vi "Global Variables.vi"() -> ()   [LabVIEW 2017]
uses:
  GRIP Contours Report.ctl
panel:
  out "Oh Crap":bool
  in  "Intake Motor Power":dbl
  in  "Intake Angle Setpoint":dbl
  in  "Intake Angle Encoder":dbl
  out "Linear Actuator Setpoint":dbl=0.6
  out "Climb?":bool
  out "Drive Gear":enum16{"Low", "High"}(ring)
  out "Elevator Gear":enum16{"Low", "High"}(ring)=enum."High"
  out "Elevator Angle":T1(ring)
  out "Elevator Position":T2(ring)
  out "Intake Hinge Position":enum16{"Up", "Down"}(ring)
  out "Setpoint":dbl=0.5
  out "Intake State":enum16{"Off", "Intake", "Spit Low", "Spit High"}(ring)
  out "Power Cube Data":T3
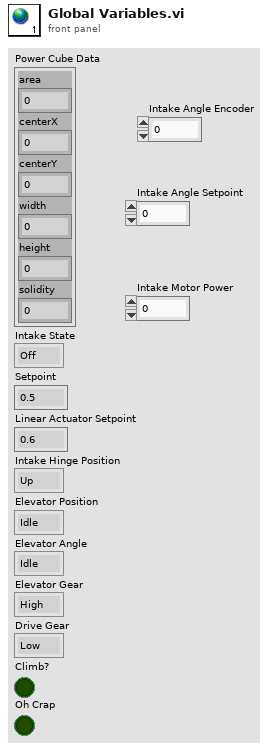
[diagram p1: front panel]
types:
  T1 = enum16{"Idle", "Portal", "Subtract", "Add", "Straight Up"}
  T2 = enum16{"Idle", "Ground", "Portal", "Switch", "Scale", "Cube Down", "Cube Up", "Add Down", "Add Up"}
  T3 = typedef "GRIP Contours Report.ctl" = cluster{"area":dbl, "centerX":dbl, "centerY":dbl, "width":dbl, "height":dbl, "solidity":dbl}
diagram:
